vi "Load and split packets from file.vi"(8 "error in":errorcluster, 11 "Path":path) -> (0 "error out":errorcluster, 1 "selected path":path, 2 "OK?":bool, 3 "Hex String":string[](array[string]))   [LabVIEW 2020]
uses:
  Globals/FPGA Globals.vi
panel:
  out "Array":string[](array[string])
  out "text":string
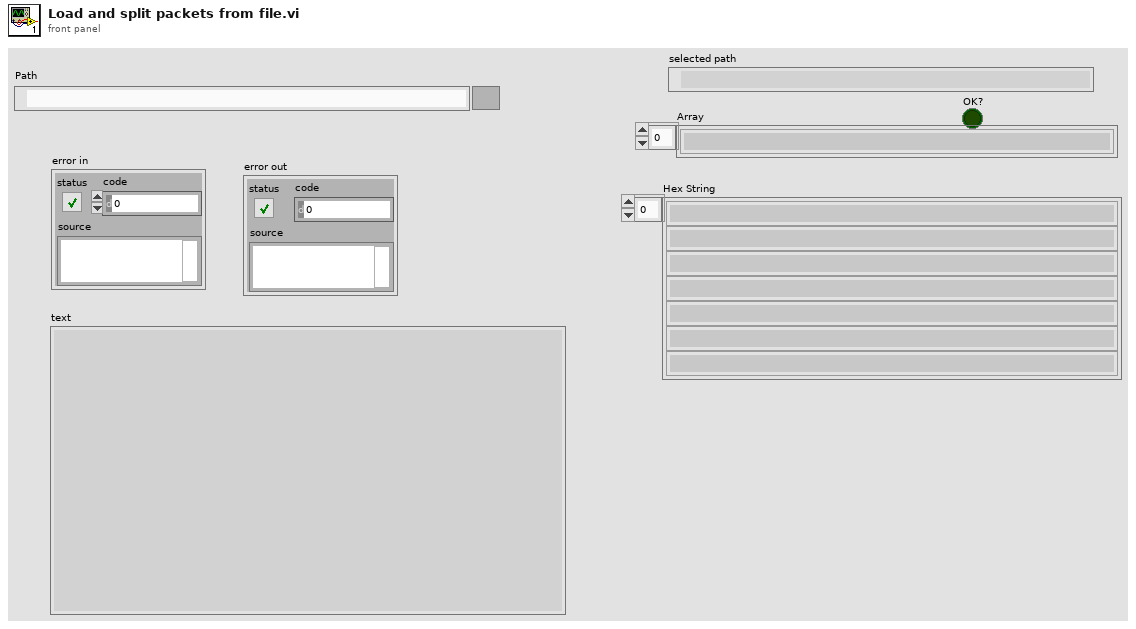
[diagram p1: front panel]
types:
  T1 = enum16{"open", "replace", "create", "open or create", "replace or create", "replace or create with confirmation"}
  T2 = typedef "FPGA Settings.ctl" = cluster{"System Clock(MHz)":dbl, "FPGA MAC 1":string, "Port Number 1":i32, "Port Number 2":i32, "FPGA MAC 2":string, "PC MAC Address":string}
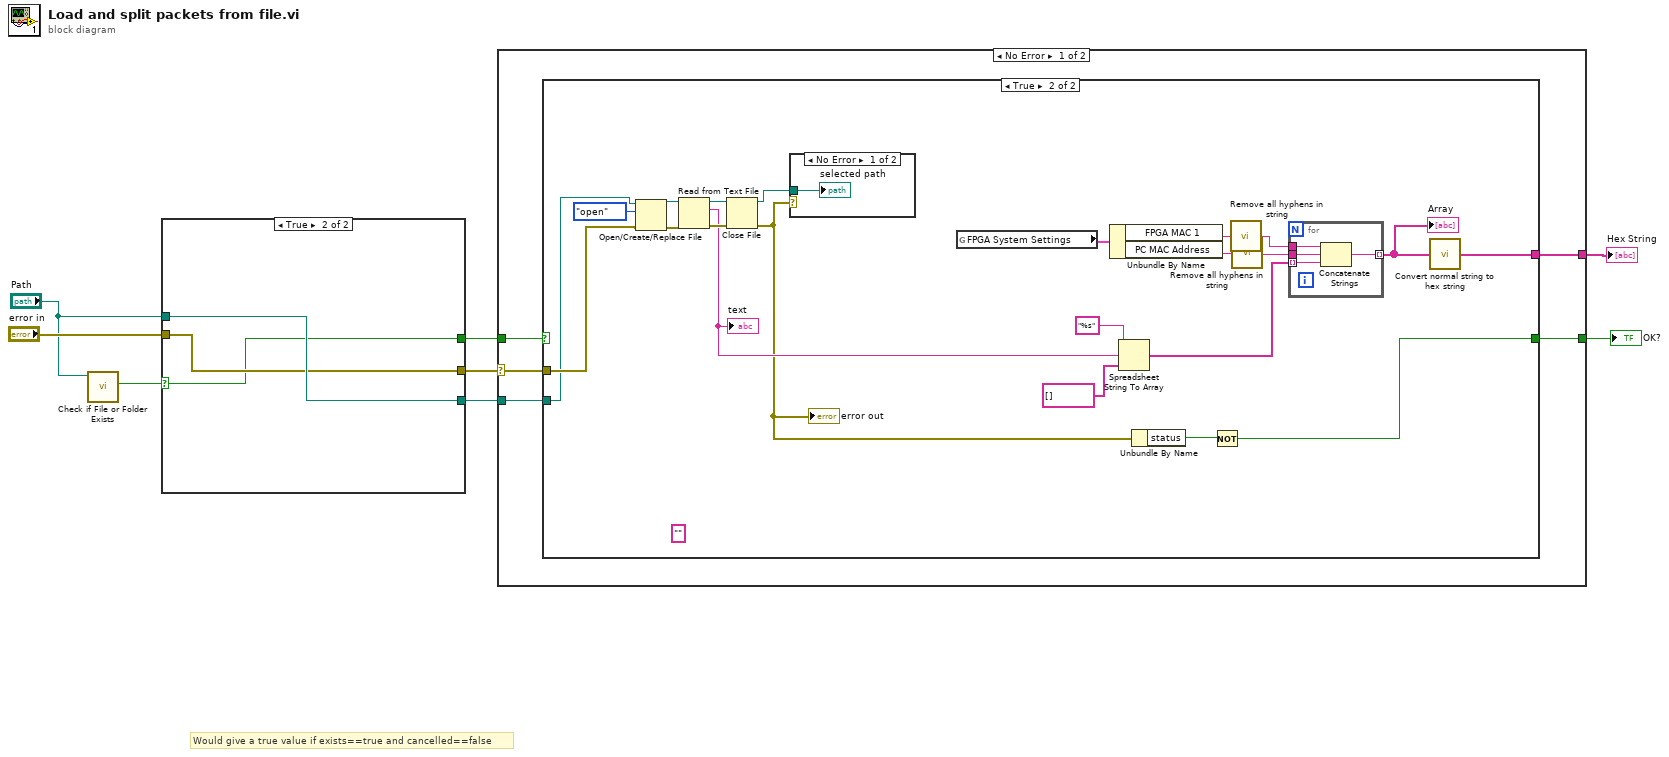
[diagram p0: block diagram]
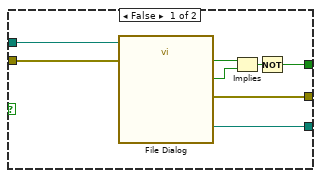
[diagram p2: hidden frame]
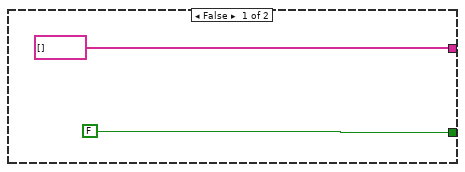
[diagram p3: hidden frame]
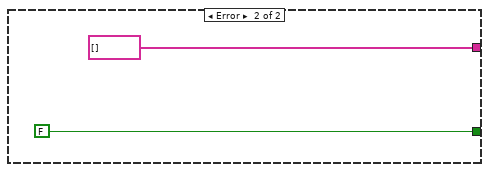
[diagram p5: hidden frame]
diagram:
  # "Would give a true value if exists==true and cancelled==false"
  n1 = call <vilib>:"Check if File or Folder Exists.vi"("path"="Path") -> ("file or folder exists?"=w1:bool)  [unwired: 8 in, 2 out]
  n2 = case shown="True" w1 {
    selector: w1 -> [_ w17]
    tunnel: "error in" -> [w16 w18]
    tunnel: [w15 w18] -> w7
    tunnel: [w11 w17] -> w6
    tunnel: [w10 w19] -> w5
    tunnel: "Path" -> [w9 w19]
    frame False {
      n3 = call "File Dialog"("start path"=w9, "error in"=w16) -> ("selected path"=w10:path, "exists"=w13:bool, "cancelled"=w12:bool, "error out"=w15:errorcluster)  [unwired: 10 in]
      n4 = Implies(1:w12, 2:w13) -> (0:w14:bool)
      n5 = Not(x=w14) -> (.not. x?=w11:bool)
    }
    frame True {
    }
  }
  n6 = case shown="No Error" w7 {
    selector: w7 -> [w23 _]
    tunnel: w6 -> [w24 _]
    tunnel: w5 -> [w22 _]
    tunnel: [w21 FALSE] -> w4
    tunnel: [w20 string[] [] ("Hex String")] -> w3
    frame No Error {
      n7 = case shown="True" w24 {
        tunnel: w23 -> [_ w43]
        tunnel: w22 -> [_ w42]
        tunnel: [FALSE w40] -> w21
        tunnel: [string[] [] ("Hex String") w29] -> w20
        frame False {
        }
        frame True {
          (unwired) ""
          n8 = Open/Create/Replace File(file path (use dialog)=w42, error in=w43, operation (0:open)=T1."open") -> (refnum out=w46:refnum<file>, error out=w47:errorcluster)  [unwired: 3 in, 1 out]
          n9 = Read from Text File(file (use dialog)=w46, error in=w47) -> (refnum out=w44:refnum<file>, text=w36:string, error out=w45:errorcluster)  [unwired: 2 in, 1 out]
          "text" <- w36
          n10 = Close File(refnum=w44, error in=w45) -> (path=w27:path, error out=w28:errorcluster)
          "error out" <- w28
          n11 = case shown="No Error" w28 {
            tunnel: w27 -> [w49 _]
            frame No Error {
              "selected path" <- w49
            }
            frame Error {
            }
          }
          n12 = global read "FPGA Globals.vi" "FPGA System Settings"() -> (w35:T2)
          n13 = Unbundle By Name(w35) -> ("FPGA MAC 1"=w34:string, "PC MAC Address"=w33:string)
          n14 = Spreadsheet String To Array(format string="%s", spreadsheet string=w36, array type (2D Dbl)=string[] []) -> (array=w37:string[])  [unwired: 1 in]
          n15 = Unbundle By Name(w28) -> ("status"=w41:bool)
          n16 = Not(x=w41) -> (.not. x?=w40:bool)
          n17 = call "Remove all hyphens in string.vi"("MAC Address"=w34) -> ("result string"=w32:string)  [unwired: 4 in]
          n18 = call "Remove all hyphens in string.vi"("MAC Address"=w33) -> ("result string"=w31:string)  [unwired: 4 in]
          n19 = for {
            tunnel: w37 -> [w53] mode=indexing
            tunnel: [w52] -> w30 mode=indexing
            tunnel: w32 -> [w51]
            tunnel: w31 -> [w50]
            n20 = Concatenate Strings(w51, w50, w53) -> (w52:string)
          }
          "Array" <- w30
          n21 = call "Convert normal string to hex string.vi"("Normal String"=w30) -> ("Hex String"=w29:string[])  [unwired: 4 in]
        }
      }
    }
    frame Error {
    }
  }
  "OK?" <- w4
  "Hex String" <- w3
